vi "Find All Strings in List.vi"(9 "List to search":string[](array[string]), 11 "String":string) -> (2 "Matches":i32[](array[numeric]))   [LabVIEW 2015]
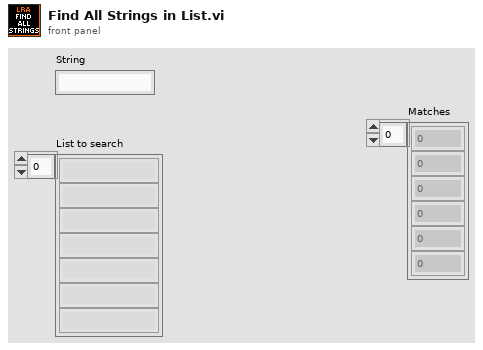
[diagram p1: front panel]
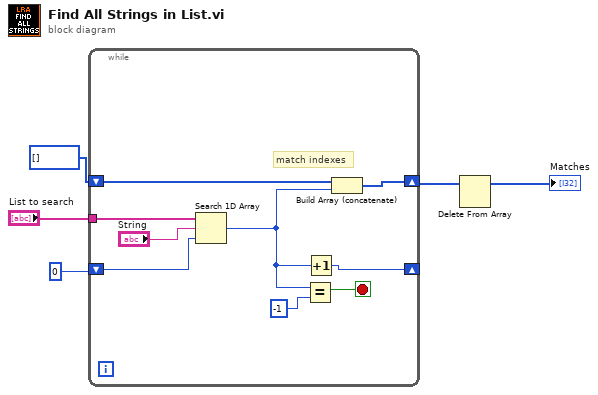
[diagram p0: block diagram]
diagram:
  n1 = while {
    shift-right: [w6] -> _
    shift-left: 0 ("index of element") -> [w12]
    shift-right: [w11] -> w2
    shift-left: i32[] [] -> [w10]
    tunnel: "List to search" -> [w13]
    stop <- w8 stop-if-true
    # "match indexes"
    n2 = Search 1D Array(1D array=w13, element="String", start index (0)=w12) -> (index of element=w7:i32)
    n3 = Equal?(x=w7, y=-1) -> (x = y?=w8:bool)
    n4 = Increment(x=w7) -> (x+1=w6:i32)
    n5 = Build Array (concatenate)(w10, w7) -> (w11:i32[])
  }
  n6 = Delete From Array(array=w2) -> (array with subset deleted=→"Matches":i32[])  [unwired: 2 in, 1 out]
